vi "Read from File.vi"(7 "Section Name":string, 8 "error in (no error)":errorcluster, 10 "INI Ref":T1, 11 "Assertion Step in":refnum<class "Assertion Step.lvclass">) -> (0 "error out":errorcluster, 2 "INI Ref out":T1, 3 "Assertion Step out":refnum<class "Assertion Step.lvclass">)   [LabVIEW 2020, in "MacroAssert.lvlib" / "Assertion Step.lvclass"]
doc: "Reads associated parameters from the file identified by <B>INI Ref</B>."
uses:
  Assertion Step.lvclass
  <vilib>/Utility/config.llb/Config Data RefNum.ctl
  <vilib>/Utility/config.llb/Read Key (String).vi
  Step/Step.lvclass
  <vilib>/Utility/config.llb/NI_LVConfig.lvlib
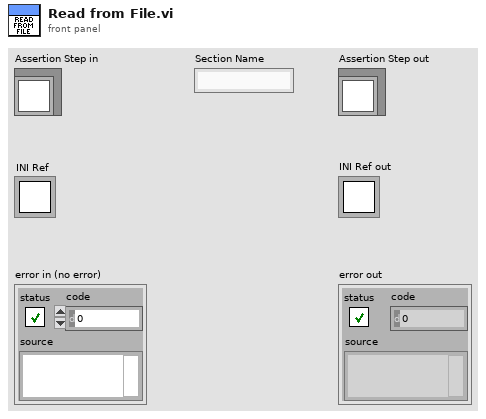
[diagram p1: front panel]
types:
  T1 = typedef "NI_LVConfig.lvlib/Config Data RefNum.ctl" = refnum<k1>
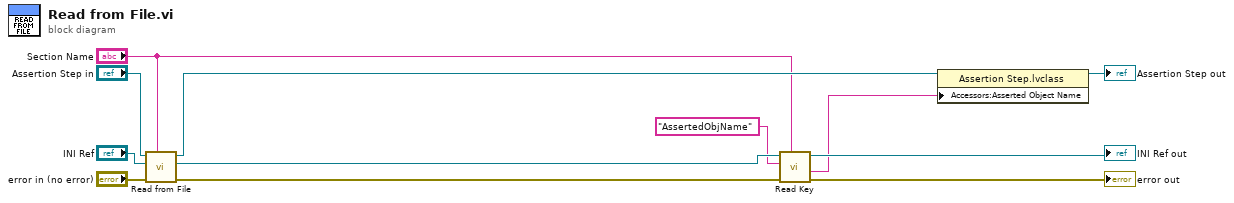
[diagram p0: block diagram]
diagram:
  n1 = call-parent "Read from File.vi"("Section Name"="Section Name", "error in (no error)"="error in (no error)", "INI Ref"="INI Ref", "Step in"="Assertion Step in") -> ("error out"=w11:errorcluster, "INI Ref out"=w8:T1, "Step out"=w5:refnum<class "Assertion Step.lvclass">)  [unwired: 5 in]
  n2 = call-poly <vilib>:"Read Key.vi"("section"="Section Name", "error in (no error)"=w11, "key"="AssertedObjName", "refnum"=w8) -> ("error out"=→"error out":errorcluster, "value"=w2:string, "refnum out"=→"INI Ref out":T1)  [unwired: 4 in, 1 out]
  n3 = property class="Assertion Step.lvclass"(reference=w5, "Accessors:Asserted Object Name"=w2) -> (reference out=→"Assertion Step out":refnum<class "Assertion Step.lvclass">)  [unwired: 1 in, 1 out]
